vi "main.vi"() -> ()   [LabVIEW 2023]
uses:
  #typedef_state.ctl
  #typedef_data.ctl
panel:
  in  "Remove":bool
  in  "ID":i32
  out "List":string[][](array[string])
  in  "Stop Button":bool
  in  "Add":bool
  in  "Manufacturer":string
  in  "Name":string
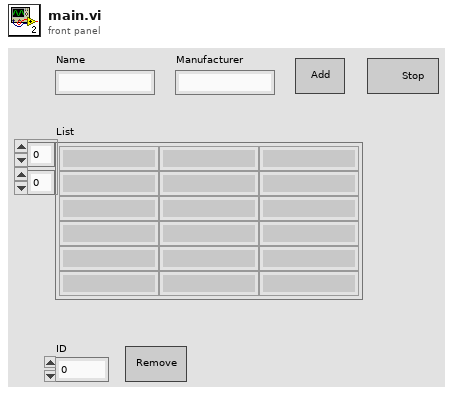
[diagram p1: front panel]
types:
  T1 = typedef "#typedef_state.ctl" = enum16{"Aplication Error", "Remove", "Add", "Stop", "Idling", "Inicializing"}
  T2 = typedef "#typedef_data.ctl" = cluster{"List":string[][], "Current ID":i32}
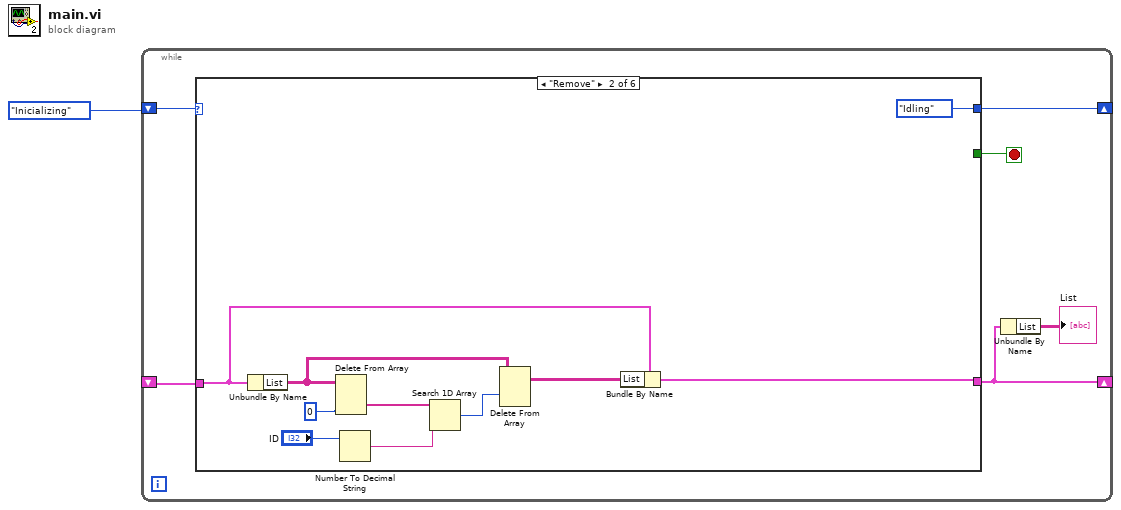
[diagram p0: block diagram]
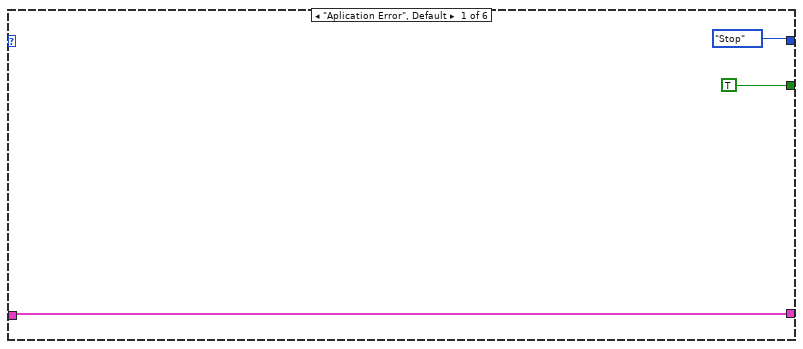
[diagram p2: hidden frame]
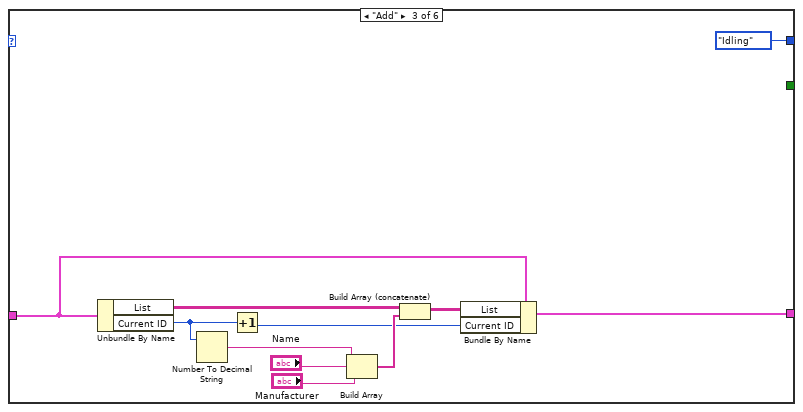
[diagram p3: hidden frame]
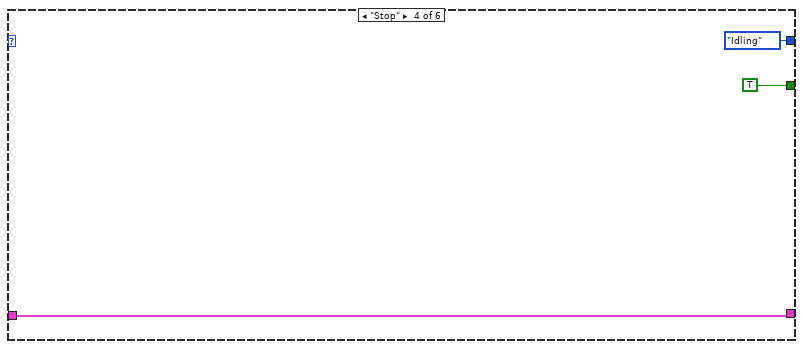
[diagram p4: hidden frame]
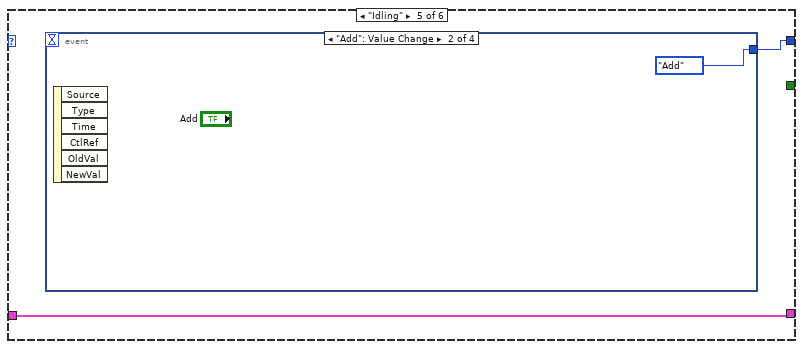
[diagram p5: hidden frame]
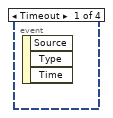
[diagram p6: hidden frame]
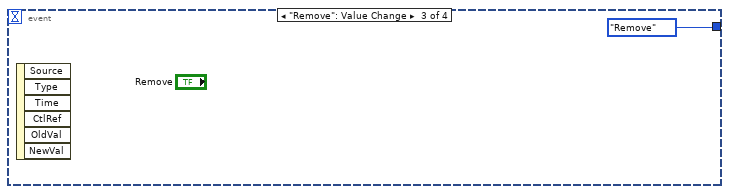
[diagram p7: hidden frame]
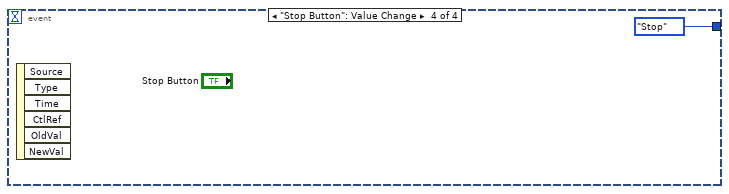
[diagram p8: hidden frame]
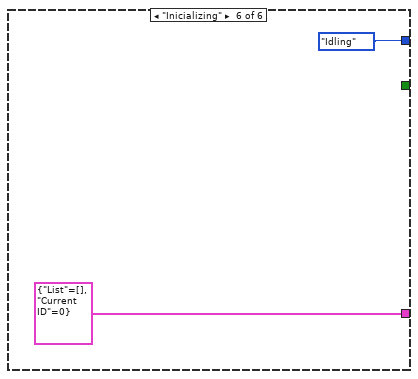
[diagram p9: hidden frame]
diagram:
  n1 = while {
    shift-right: [w4] -> _
    shift-left: _ -> [w6]
    shift-right: [w5] -> _
    shift-left: #typedef_state."Inicializing" ("State") -> [w7]
    stop <- w2 stop-if-true
    n2 = case shown="\"Remove\"" w7 {
      tunnel: [w9 w11 w21 w34 w36 T2 {"List"=[], "Current ID"=0} ("Cluster")] -> w4
      tunnel: w6 -> [w9 w13 w24 w34 w36 _]
      tunnel: [#typedef_state."Stop" ("State") #typedef_state."Idling" ("State") #typedef_state."Idling" ("State") #typedef_state."Idling" ("State") w35 #typedef_state."Idling" ("State")] -> w5
      tunnel: [TRUE _ _ TRUE _ _] -> w2
      frame "Aplication Error", Default {
      }
      frame "Remove" {
        n3 = Unbundle By Name(w13) -> ("List"=w15:string[][])
        n4 = Delete From Array(array=w15, index (col)=0) -> (deleted portion=w17:string[])  [unwired: 2 in, 1 out]
        n5 = Number To Decimal String(number="ID") -> (decimal integer string=w16:string)  [unwired: 1 in]
        n6 = Search 1D Array(1D array=w17, element=w16) -> (index of element=w14:i32)  [unwired: 1 in]
        n7 = Delete From Array(array=w15, index (row)=w14) -> (array with subset deleted=w12:string[][])  [unwired: 2 in, 1 out]
        n8 = Bundle By Name(cluster=w13, "List"=w12) -> (w11:T2)
      }
      frame "Add" {
        n9 = Unbundle By Name(w24) -> ("List"=w26:string[][], "Current ID"=w28:i32)
        n10 = Number To Decimal String(number=w28) -> (decimal integer string=w27:string)  [unwired: 1 in]
        n11 = Increment(x=w28) -> (x+1=w23:i32)
        n12 = Build Array(w27, "Name", "Manufacturer") -> (w25:string[])
        n13 = Build Array (concatenate)(w26, w25) -> (w22:string[][])
        n14 = Bundle By Name(cluster=w24, "List"=w22, "Current ID"=w23) -> (w21:T2)
      }
      frame "Stop" {
      }
      frame "Idling" {
        n15 = event shown="[1] \"Add\": Value Change" {
          selector: _ -> [_ _ _ _]
          dyn-events: _ -> [_ _ _ _]
          timeout: _ -> [_ _ _ _]
          tunnel: [_ #typedef_state."Add" ("State") #typedef_state."Remove" ("State") #typedef_state."Stop" ("State")] -> w35
          event Timeout {
            n16 = event-data() -> ()  [unwired: 1 in, 3 out]
          }
          event "Add": Value Change {
            n17 = event-data() -> ()  [unwired: 1 in, 6 out]
          }
          event "Remove": Value Change {
            n18 = event-data() -> ()  [unwired: 1 in, 6 out]
          }
          event "Stop Button": Value Change {
            n19 = event-data() -> ()  [unwired: 1 in, 6 out]
          }
        }
      }
      frame "Inicializing" {
      }
    }
    n20 = Unbundle By Name(w4) -> ("List"=→"List":string[][])
  }
